vi "Gen_Fault_Dataset.vi"(7 "Norm fctor":sgl=400.0, 9 "Number of Samples Per Class":i32=5000, 11 "Dataset Folder Path":path) -> (3 "Dataset Folder Path":path)   [LabVIEW 2020]
uses:
  <vilib>/Utility/file.llb/Write Delimited Spreadsheet (DBL).vi
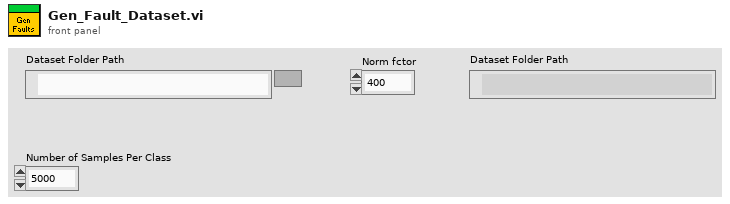
[diagram p1: front panel]
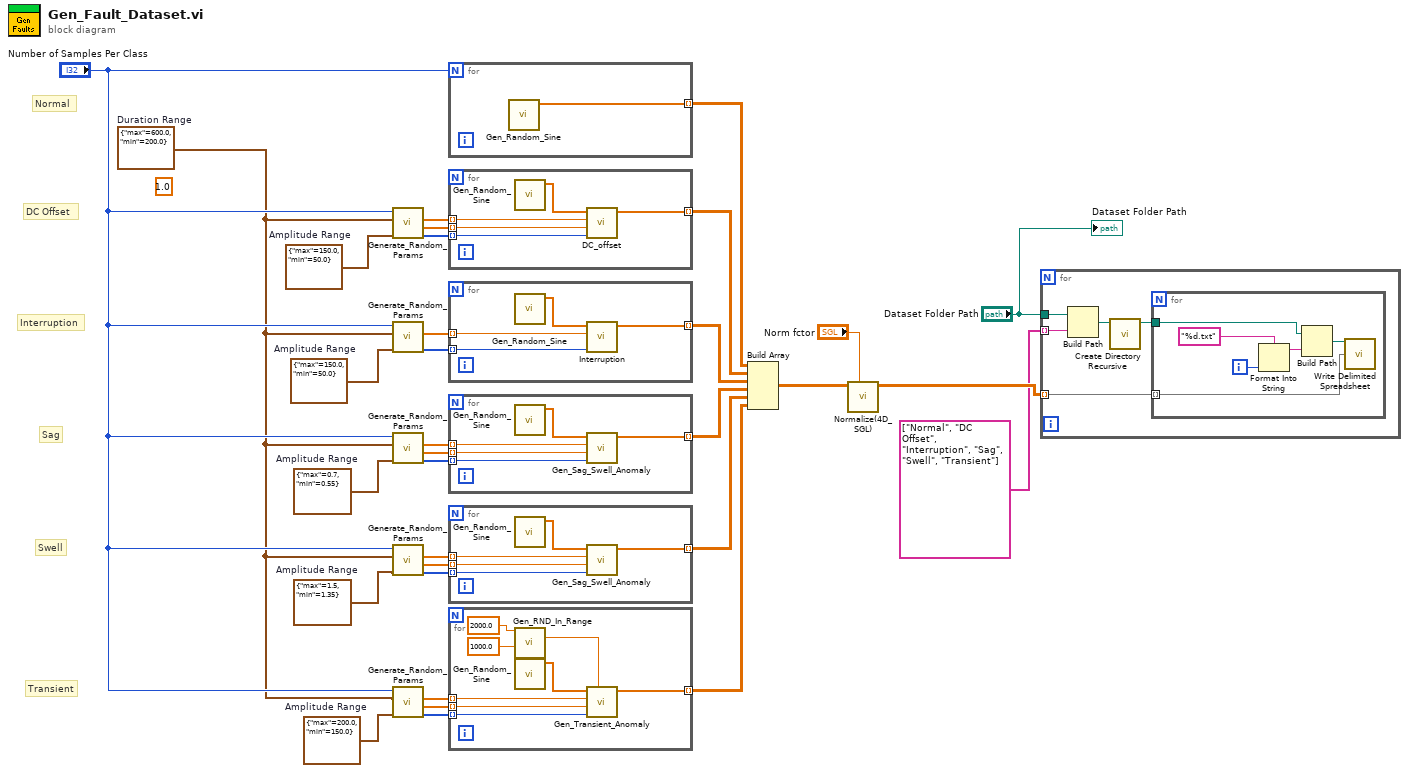
[diagram p0: block diagram]
diagram:
  w2 = cluster{"max":dbl, "min":dbl} {"max"=150.0, "min"=50.0}  # Amplitude Range
  (unwired) 1.0
  w9 = cluster{"max":dbl, "min":dbl} {"max"=200.0, "min"=150.0}  # Amplitude Range
  w10 = cluster{"max":dbl, "min":dbl} {"max"=1.5, "min"=1.35}  # Amplitude Range
  w11 = cluster{"max":dbl, "min":dbl} {"max"=0.7, "min"=0.55}  # Amplitude Range
  w6 = cluster{"max":dbl, "min":dbl} {"max"=600.0, "min"=200.0}  # Duration Range
  w12 = cluster{"max":dbl, "min":dbl} {"max"=150.0, "min"=50.0}  # Amplitude Range
  # "Normal"
  # "Swell"
  # "DC Offset"
  # "Interruption"
  # "Sag"
  # "Transient"
  n1 = call "Generate_Random_Params.vi"("Amplitude Range"=w12, "Duration Range"=w6, "Samples"="Number of Samples Per Class") -> ("Duration"=w19:i32[], "Amplitude"=w20:dbl[], "Position"=w21:dbl[])  [unwired: 6 in]
  n2 = call "Generate_Random_Params.vi"("Amplitude Range"=w2, "Duration Range"=w6, "Samples"="Number of Samples Per Class") -> ("Duration"=w23:i32[], "Position"=w24:dbl[])  [unwired: 6 in, 1 out]
  n3 = call "Generate_Random_Params.vi"("Amplitude Range"=w11, "Duration Range"=w6, "Samples"="Number of Samples Per Class") -> ("Duration"=w28:i32[], "Amplitude"=w27:dbl[], "Position"=w26:dbl[])  [unwired: 6 in]
  n4 = call "Generate_Random_Params.vi"("Amplitude Range"=w10, "Duration Range"=w6, "Samples"="Number of Samples Per Class") -> ("Duration"=w29:i32[], "Amplitude"=w30:dbl[], "Position"=w31:dbl[])  [unwired: 6 in]
  n5 = call "Generate_Random_Params.vi"("Amplitude Range"=w9, "Duration Range"=w6, "Samples"="Number of Samples Per Class") -> ("Duration"=w14:i32[], "Amplitude"=w13:dbl[], "Position"=w16:dbl[])  [unwired: 6 in]
  n6 = for {
    N: "Number of Samples Per Class" -> [_]
    tunnel: [w33] -> w17 mode=indexing
    n7 = call "Gen_Random_Sine.vi"() -> ("data"=w33:sgl[])  [unwired: 11 in]
  }
  n8 = for {
    tunnel: [w38] -> w18 mode=indexing
    tunnel: w21 -> [w37] mode=indexing
    tunnel: w20 -> [w36] mode=indexing
    tunnel: w19 -> [w35] mode=indexing
    n9 = call "Gen_Random_Sine.vi"() -> ("data"=w34:sgl[])  [unwired: 11 in]
    n10 = call "DC_offset.vi"("Duration"=w35, "Ampltude"=w36, "Position"=w37, "Sine"=w34) -> ("Sine+Anomaly"=w38:sgl[])  [unwired: 7 in]
  }
  n11 = for {
    tunnel: [w42] -> w22 mode=indexing
    tunnel: w24 -> [w41] mode=indexing
    tunnel: w23 -> [w40] mode=indexing
    n12 = call "Gen_Random_Sine.vi"() -> ("data"=w39:sgl[])  [unwired: 11 in]
    n13 = call "Interruption.vi"("Duration"=w40, "Position"=w41, "Sine"=w39) -> ("Sine+Anomaly"=w42:sgl[])  [unwired: 8 in]
  }
  n14 = for {
    tunnel: [w47] -> w25 mode=indexing
    tunnel: w26 -> [w46] mode=indexing
    tunnel: w27 -> [w45] mode=indexing
    tunnel: w28 -> [w44] mode=indexing
    n15 = call "Gen_Random_Sine.vi"() -> ("data"=w43:sgl[])  [unwired: 11 in]
    n16 = call "Gen_Sag_Swell_Anomaly.vi"("Duration"=w44, "Amplitude"=w45, "Position"=w46, "Sine"=w43) -> ("Sine+Anomaly"=w47:sgl[])  [unwired: 7 in]
  }
  n17 = for {
    tunnel: [w52] -> w32 mode=indexing
    tunnel: w31 -> [w51] mode=indexing
    tunnel: w30 -> [w50] mode=indexing
    tunnel: w29 -> [w49] mode=indexing
    n18 = call "Gen_Random_Sine.vi"() -> ("data"=w48:sgl[])  [unwired: 11 in]
    n19 = call "Gen_Sag_Swell_Anomaly.vi"("Duration"=w49, "Amplitude"=w50, "Position"=w51, "Sine"=w48) -> ("Sine+Anomaly"=w52:sgl[])  [unwired: 7 in]
  }
  n20 = for {
    tunnel: [w60] -> w8 mode=indexing
    tunnel: w16 -> [w59] mode=indexing
    tunnel: w14 -> [w57] mode=indexing
    tunnel: w13 -> [w53] mode=indexing
    n21 = call "Gen_RND_In_Range.vi"("Upper Bound"=2000.0 ("frequency"), "Lower Bound"=1000.0 ("Variation%")) -> ("RND_In_Range"=w54:dbl)  [unwired: 13 in]
    n22 = call "Gen_Random_Sine.vi"() -> ("data"=w58:sgl[])  [unwired: 11 in]
    n23 = call "Gen_Transient_Anomaly.vi"("Frequency"=w54, "Tau"=w57, "Amplitude"=w53, "Position"=w59, "Sine"=w58) -> ("Sine+Anomaly"=w60:sgl[])  [unwired: 6 in]
  }
  n24 = Build Array(w17, w18, w22, w25, w32, w8) -> (w7:sgl[][][])
  n25 = call "Normalize(4D_SGL).vi"("Norm Factor"="Norm fctor", "Data In"=w7) -> ("Normalized Out"=w5:sgl[][][])  [unwired: 9 in]
  n26 = for {
    tunnel: w5 -> [w65] mode=indexing
    tunnel: "Dataset Folder Path" -> [w64]
    tunnel: string[] ["Normal", "DC Offset", "Interruption", "Sag", "Swell", "Transient"] -> [w62] mode=indexing
    n27 = Build Path(base path=w64, name or relative path=w62) -> (appended path=w63:path)
    n28 = call <vilib>:"Create Directory Recursive.vi"("directory"=w63) -> ("directory copy"=w61:path)  [unwired: 4 in, 2 out]
    n29 = for {
      tunnel: w65 -> [w70] mode=indexing
      tunnel: w61 -> [w71]
      i -> [w67]
      n30 = Format Into String(format string="%d.txt", w67) -> (resulting string=w66:string)  [unwired: 2 in, 1 out]
      n31 = Build Path(base path=w71, name or relative path=w66) -> (appended path=w69:path)
      n32 = call-poly <vilib>:"Write Delimited Spreadsheet.vi"("file path (dialog if empty)"=w69, "1D data"=w70) -> ()  [unwired: 12 in, 2 out]
    }
  }
  "Dataset Folder Path" <- "Dataset Folder Path"
